vi "Restart.vi"(8 "error in (no error)":errorcluster, 11 "Output Actor Hardware Interface in":refnum<class "Output Actor Hardware Interface.lvclass">) -> (0 "error out":errorcluster, 3 "Output Actor Hardware Interface out":refnum<class "Output Actor Hardware Interface.lvclass">)   [LabVIEW 2015, in "Output Actor Hardware Interface.lvclass"]
uses:
  Output Actor Hardware Interface.lvclass
  Output Actor/Output Actor Interface/Output Actor Interface.lvclass/Output Actor Interface.ctl
  <vilib>/ActorFramework/Message Enqueuer/Message Enqueuer.lvclass/Message Enqueuer.ctl
  <vilib>/ActorFramework/Message Enqueuer/Enqueue.vi
  <vilib>/ActorFramework/Message Priority Queue/Priority Enqueue.vi
  <vilib>/ActorFramework/Message Enqueuer/Message Enqueuer.lvclass
  Output Actor Hardware Messages/Do Deinitialize Msg/Do Deinitialize Msg.lvclass
  Output Actor/Output Actor Interface/Output Actor Interface.lvclass
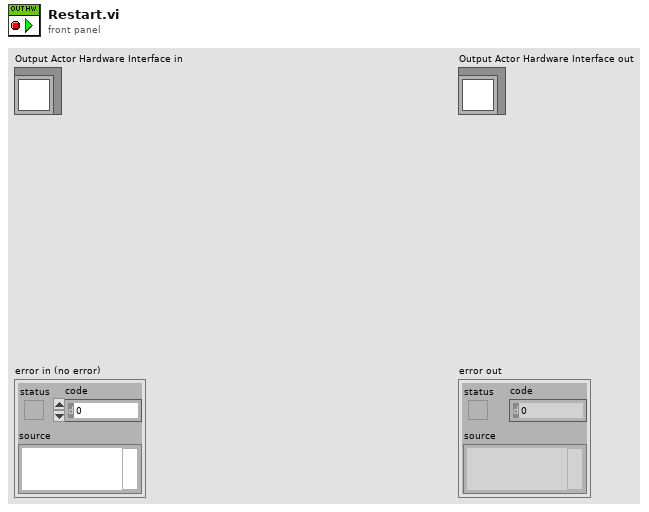
[diagram p1: front panel]
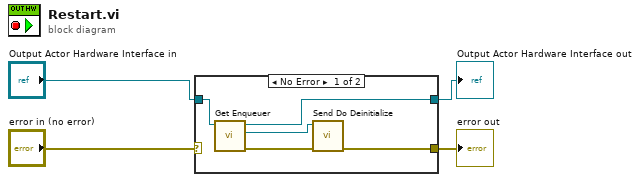
[diagram p0: block diagram]
diagram:
  n1 = case shown="No Error" "error in (no error)" {
    selector: "error in (no error)" -> [_ w11]
    tunnel: [w5 w11] -> w3
    tunnel: [w8 w10] -> w1
    tunnel: "Output Actor Hardware Interface in" -> [w9 w10]
    frame No Error {
      n2 = call "Get Enqueuer.vi"("Output Actor Interface in"=w9) -> ("error out"=w6:errorcluster, "Actor Framework:Message Enqueuer"=w7:refnum<class "Message Enqueuer.lvclass">, "Output Actor Interface out"=w8:refnum<class "Output Actor Hardware Interface.lvclass">)  [unwired: 8 in]
      n3 = call "Send Do Deinitialize.vi"("error in (no error)"=w6, "Message Enqueuer"=w7) -> ("error out"=w5:errorcluster)  [unwired: 8 in, 1 out]
    }
    frame Error {
    }
  }
  "error out" <- w3
  "Output Actor Hardware Interface out" <- w1
